vi "Clicking SubVi.vi"(10 "Numeric":i32, 11 "Coords":T1) -> (3 "Array":cluster{"Horizontal":i32, i32}[](array[cluster]))   [LabVIEW 2014]
uses:
  <vilib>/Utility/miscctls.llb/LVPoint32TypeDef.ctl
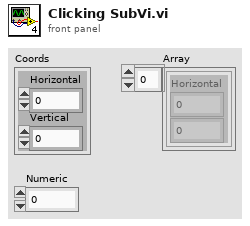
[diagram p1: front panel]
types:
  T1 = typedef "LVPoint32TypeDef.ctl" = cluster{"Horizontal":i32, "Vertical":i32}
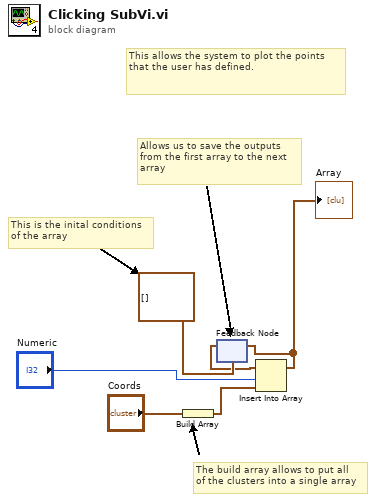
[diagram p0: block diagram]
diagram:
  # "This allows the system to plot the points \nthat the user has defined."
  # "The build array allows to put all \nof the clusters into a single array"
  # "This is the inital conditions\nof the array"
  # "Allows us to save the outputs\nfrom the first array to the next \narray"
  n1 = Build Array("Coords") -> (w1:T1[])
  n2 = feedback #1(cluster{"Horizontal":i32, i32}[] []) -> (w3:cluster{"Horizontal":i32, i32}[])
  n3 = Insert Into Array(array=w3, index="Numeric", new element=w1) -> (w6:cluster{"Horizontal":i32, i32}[])
  "Array" <- w6
  n4 = feedback-in #1(w6) -> ()
